vi "IsErrorTypeTunnel__slk_mt.vi"(8 "error in (no error)":errorcluster, 11 "tunnel refnum in":refnum<vi>) -> (0 "error out":errorcluster, 2 "error type tunnel?":bool, 3 "duplicated tunnel refnum out":refnum<vi>)   [LabVIEW 2013, in "Lazyboots Menu Tool.lvlib"]
doc: "Checks if the tunnel type is error."
uses:
  Library/Lazyboots Menu Tool.lvlib
panel:
  # "IsErrorTypeTunnel__slk_mt.vi\nChecks if the tunnel type is error.\n\nNOTICE -- YOU MUST LEAVE THIS NOTICE IN PLACE.\n\nCopyright (c) 2011, LIANG LIU Shawn.Liu.cn@gmail.com\nAll rights reserved.\n\nRedistribution and use in source and binary forms, with or without modification, are permitted provided that the following conditions are met:\n-Redistributions of source code must retain the above copyright notice, this list of conditions and the following disclaimer.\n-Redistributions in binary form must reproduce the above copyright notice, this list of conditions and the following disclaimer in the documentation and/or other materials provided with the distribution.\n-Neither the name of the eLp nor the names of its contributors may be used to endorse or promote products derived from this software without specific prior written permission.\n\nTHIS SOFTWARE IS PROVIDED BY THE COPYRIGHT HOLDERS AND CONTRIBUTORS \"AS IS\" AND ANY EXPRESS OR IMPLIED WARRANTIES, INCLUDING, BUT NOT LIMITED TO, THE IMPLIED WARRANTIES OF MERCHANTABILITY AND FITNESS FOR A PARTICULAR PURPOSE ARE DISCLAIMED. IN NO EVENT SHALL THE COPYRIGHT HOLDER OR CONTRIBUTORS BE LIABLE FOR ANY DIRECT, INDIRECT, INCIDENTAL, SPECIAL, EXEMPLARY, OR CONSEQUENTIAL DAMAGES (INCLUDING, BUT NOT LIMITED TO, PROCUREMENT OF SUBSTITUTE GOODS OR SERVICES; LOSS OF USE, DATA, OR PROFITS; OR BUSINESS INTERRUPTION) HOWEVER CAUSED AND ON ANY THEORY OF LIABILITY, WHETHER IN CONTRACT, STRICT LIABILITY, OR TORT (INCLUDING NEGLIGENCE OR OTHERWISE) ARISING IN ANY WAY OUT OF THE USE OF THIS SOFTWARE, EVEN IF ADVISED OF THE POSSIBILITY OF SUCH DAMAGE."
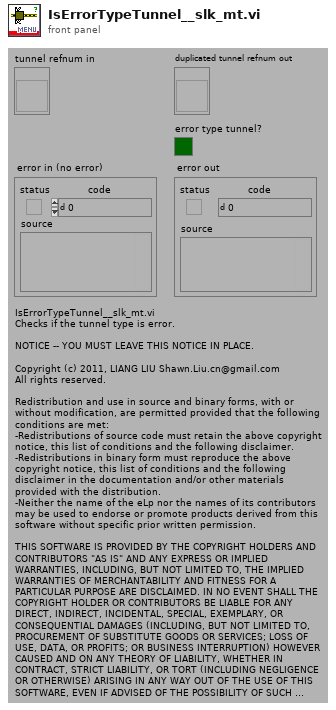
[diagram p1: front panel]
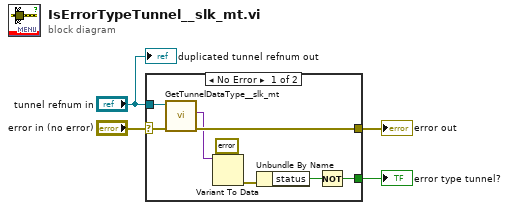
[diagram p0: block diagram]
diagram:
  n1 = case shown="No Error" "error in (no error)" {
    selector: "error in (no error)" -> [w8 w14]
    tunnel: [w9 FALSE] -> w4
    tunnel: [w6 w14] -> w3
    tunnel: "tunnel refnum in" -> [w7 _]
    frame No Error {
      n2 = call "GetTunnelDataType__slk_mt.vi"("error in (no error)"=w8, "tunnel refnum in"=w7) -> ("error out"=w6:errorcluster, "data type"=w5:variant)  [unwired: 7 in, 1 out]
      n3 = Variant To Data(type=errorcluster {"status"=FALSE, "code"=0, "source"=""} ("error out"), Variant=w5) -> (error out=w11:errorcluster)  [unwired: 1 in, 1 out]
      n4 = Unbundle By Name(w11) -> ("status"=w10:bool)
      n5 = Not(x=w10) -> (.not. x?=w9:bool)
    }
    frame Error {
    }
  }
  "error type tunnel?" <- w4
  "error out" <- w3
  "duplicated tunnel refnum out" <- "tunnel refnum in"
